vi "CC WebRelay Set.vi"(8 "error in (no error)":errorcluster, 9 "state":bool, 10 "Relay (1 to 10)":i32=1 min=1 max=10 step=1, 11 "connection ID":refnum<k5>) -> (0 "error out":errorcluster, 3 "connection ID out":refnum<k5>)   [LabVIEW 2021]
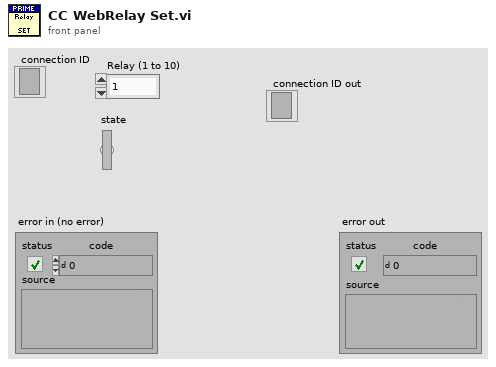
[diagram p1: front panel]
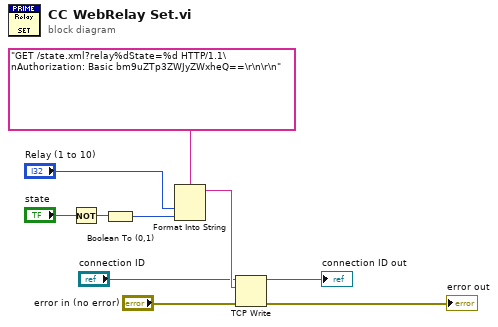
[diagram p0: block diagram]
diagram:
  n1 = Not(x="state") -> (.not. x?=w4:bool)
  n2 = Boolean To (0,1)(Boolean=w4) -> (0, 1=w2:i16)
  n3 = Format Into String(format string="GET /state.xml?relay%dState=%d HTTP/1.1\nAuthorization: Basic bm9uZTp3ZWJyZWxheQ==\r\n\r\n", "Relay (1 to 10)", w2) -> (resulting string=w9:string)  [unwired: 2 in, 1 out]
  n4 = TCP Write(connection ID="connection ID", data in=w9, error in (no error)="error in (no error)") -> (connection ID out=→"connection ID out":refnum<k5>, error out=→"error out":errorcluster)  [unwired: 1 in, 1 out]
